vi "Toggle3.vi"(10 "ForceOff3":bool, 11 "Input3":bool) -> (2 "Output3":bool)   [LabVIEW 2020]
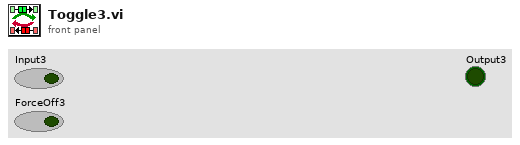
[diagram p1: front panel]
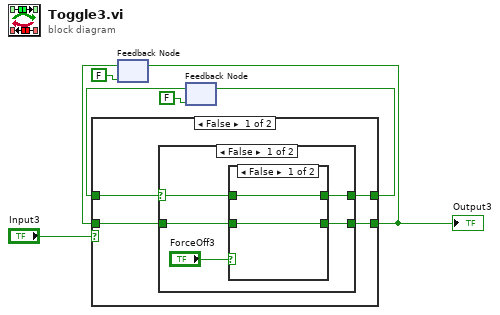
[diagram p0: block diagram]
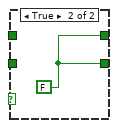
[diagram p2: hidden frame]
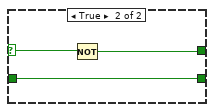
[diagram p3: hidden frame]
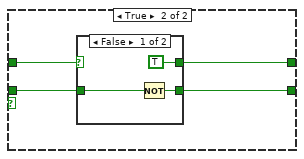
[diagram p4: hidden frame]
diagram:
  n1 = feedback #1(FALSE) -> (w6:bool)
  n2 = feedback #2(FALSE) -> (w4:bool)
  n3 = case shown="False" "Input3" {
    tunnel: [w11 w25] -> w2
    tunnel: w6 -> [w8 w26]
    tunnel: w4 -> [w10 w24]
    tunnel: [w9 w23] -> w3
    frame False {
      n4 = case shown="False" w10 {
        selector: w10 -> [w13 w22]
        tunnel: [w15 w20] -> w11
        tunnel: [w14 w21] -> w9
        tunnel: w8 -> [w12 w20]
        frame False {
          n5 = case shown="False" "ForceOff3" {
            tunnel: [w17 w19] -> w15
            tunnel: [w18 w19] -> w14
            tunnel: w13 -> [w18 _]
            tunnel: w12 -> [w17 _]
            frame False {
            }
            frame True {
              w19 = FALSE
            }
          }
        }
        frame True {
          n6 = Not(x=w22) -> (.not. x?=w21:bool)
        }
      }
    }
    frame True {
      n7 = case shown="False" w24 {
        selector: w24 -> [_ w30]
        tunnel: w26 -> [w28 w31]
        tunnel: [w29 w31] -> w25
        tunnel: [TRUE w30] -> w23
        frame False {
          n8 = Not(x=w28) -> (.not. x?=w29:bool)
        }
        frame True {
        }
      }
    }
  }
  "Output3" <- w2
  n9 = feedback-in #1(w2) -> ()
  n10 = feedback-in #2(w3) -> ()
